vi "Boolean to String.vi"(7 "Boolean":bool) -> (8 "Boolean String":string)   [LabVIEW 2010]
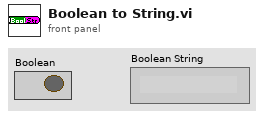
[diagram p1: front panel]
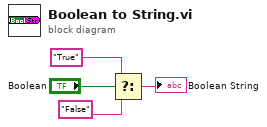
[diagram p0: block diagram]
diagram:
  n1 = Select(t="True" ("Boolean String"), s="Boolean", f="False" ("Boolean String")) -> (s? t:f=→"Boolean String":string)
